vi "Close.vi"(0 "Data In":T2={"Console log"="", "GUI_Events"={"To_GUI-Producer"=refnum, "To_GUI-Error_message"=refnum, "To_GUI-msg_list"=refnum, "To_GUI-Session"=refnum, "To_GUI-Pre-Session"=refnum, "To_GUI-Consumer"=refnum}, "Function_Queue"={"Queue_MIDI_Handler"=refnum, "Queue_Session"=refnum, "Queue_Producer"=refnum, "Queue_Consumer"=refnum}, "Timout-Time[ms]"=0, "MIDI-Messages"=[], "Com Session State"=enum."Active Session", "Result Data"={"Diff"=[], "Tx Byte"=[], "Rx Byte"=[], "Send Log"=[], "Parsed Data"={"Tx MIDI Tag"=[], "Tx MIDI Parsed Data"=[], "Tx Error"=[], "Tx Running States"=[], "Rx MIDI Tag"=[], "Rx MIDI Parsed Data"=[], "Rx Error"=[], "Rx Running States"=[], "Diff"=[]}}, "Get #"=[], "CPU(ms)"=0}, 11 "Error In":errorcluster, 12 "MIDI Data":T19, 13 "Consumer Data":T15={"Queue_Consumer"=refnum, "Selected Consumer"=enum."Random", "Session Data"={"Tx-Data"=[], "Rx-Data"=[], "MIDI-Message log"=[{"Message Name"="", "Meta value"=0, "Datastring"="", "Datatype"=enum."No Data"}]}, "Timout-Time[ms]"=0, "To_GUI-Consumer"=refnum, "CPU(ms)"=0, "Console log"="", "MIDI Parse Data"={"MIDI-Bytes In"=[145, 60, 100], "MIDI Tag"=[], "MIDI Parsed Data"=[], "Iteration"=0, "Error?"=[], "Running States"=[], "Running Statusbyte"=0, "Running StatusString"="", "Third Byte Flag"=FALSE, "Current Byte"=0, "Sysex"="", "Expect Databyte"=FALSE}, "Session Inspection Data"={"Diff"=[], "Tx Byte"=[], "Rx Byte"=[], "Send Log"=[], "Parsed Data"={"Tx MIDI Tag"=[], "Tx MIDI Parsed Data"=[], "Tx Error"=[], "Tx Running States"=[], "Rx MIDI Tag"=[], "Rx MIDI Parsed Data"=[], "Rx Error"=[], "Rx Running States"=[], "Diff"=[]}}} {"MIDI Parse Data"."Current Byte" format="%.0x"; "MIDI Parse Data"."Running Statusbyte" format="%.0x"; "MIDI Parse Data"."MIDI-Bytes In" format="%.0x"}, 14 "Producer-Data":T11={"Queue_Producer"=refnum, "Queue_Consumer"=refnum, "To_GUI-Error_message"=refnum, "Rx-Data"=[], "Tx-Data"=[], "Console log"="", "Communication Settings"={"Tx Protocol"=enum."Not Active", "Rx Protocol"=enum."Serial", "Serial"={"Tx Port"="", "Rx Port"="", "Baud rate"=31250, "Parity"=enum."Space", "Data bits"=8, "Stop bits"=10, "Flow control"=enum."None", "Tx Resource"="", "Rx Resource"=""}, "MIDI Device"={"Input uDevice ID"=0, "Output uDevice ID"=0, "hmidiout Handle"=0, "hmidiin Handle"=0}, "Bluetooth"={"Dummy"=""}, "USB"={"Dummy"=""}}, "MIDI-Messages"=[], "Queue_Session"=refnum, "To_GUI-Pre-Session"=refnum, "To_GUI-Producer"=refnum, "Tx Info"={"Datatype"=[], "Bytesize"=[], "Strings"=[], "ByteSum"=0}, "Payload"=variant, "Timout-Time[ms]"=0, "To_GUI-Session"=refnum, "CPU(ms)"=0}) -> (15 "Error Out":errorcluster)   [LabVIEW 2019]
doc: "Closing of the software:\n- Storing console entries for debugging."
uses:
  Common/Controls/Application_Data.ctl
  Common/Controls/App_Events.ctl
  Common/Controls/App_Queues.ctl
  Common/Controls/Application_Message.ctl
  Common/Controls/Application_State.ctl
  MIDI/Controls/MIDI-Message_Array.ctl
  MIDI/Controls/MIDI-Message_Cluster.ctl
  MIDI/Controls/Meta_Commands.ctl
  Producer/Controls/Session_State.ctl
  Consumer/Controls/Consumer_Result.ctl
  Consumer/Controls/Parsed_Data.ctl
  Producer/Controls/Producer-Data.ctl
  Common/Controls/Communication_Settings.ctl
  Common/Controls/Communication_Protocols.ctl
  Producer/Controls/Prod - Tx_Info.ctl
  Consumer/Controls/Consumer_Data.ctl
  Consumer/Controls/Consumer_States.ctl
  Consumer/Controls/Transfer_Data.ctl
  Consumer/Controls/Parser-data.ctl
  MIDI/Controls/MIDI-Data.ctl
  <vilib>/Utility/error.llb/DialogType.ctl
  86581a33-42cb-4fee-adae-e4a703b4ff76.vi
  <vilib>/Array/Sort 2D Array - Pop Stack.vi
  <vilib>/Array/Sort 2D Array - Push Stack.vi
panel:
  in  "Tab Control":T1(tab)
  out "Final Console":string
  out "Error Message":string
  out "VI-filename":string
  out "VI Path":path
  in  "Tabs Visible?":bool
  in  "Tool Bar:Visible":bool
  out "Revision Number":u32
  out "VI-Name":string
  # "Settings"
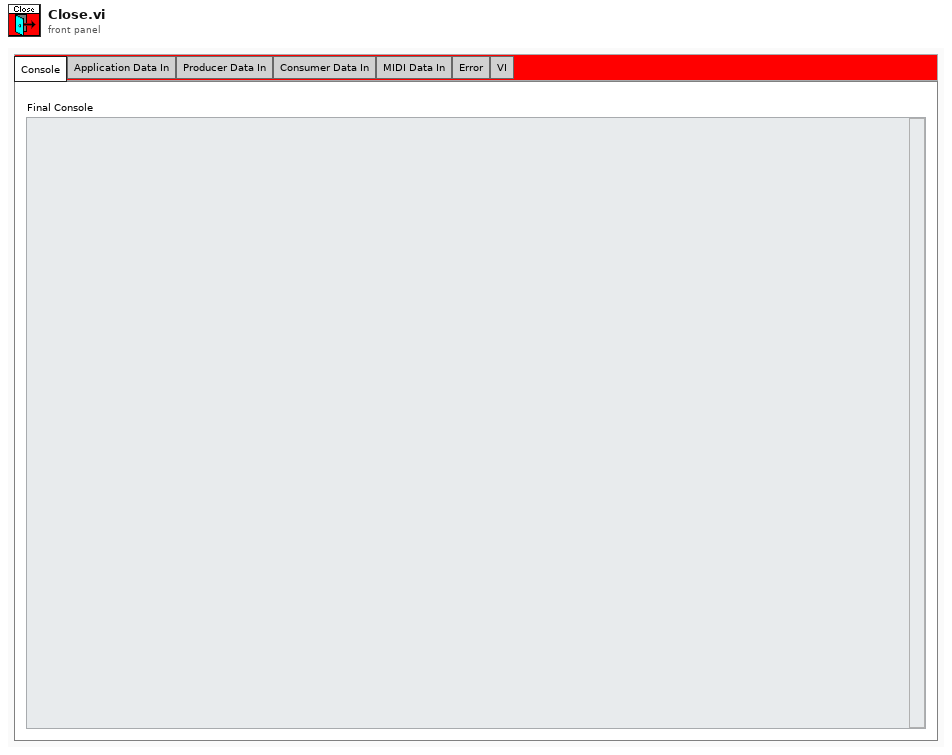
[diagram p1: front panel]
types:
  T1 = enum32{"Console", "Application Data In", "Producer Data In", "Consumer Data In", "MIDI Data In", "Error", "VI"}
  T2 = typedef "Application_Data.ctl" = cluster{"Console log":string, "GUI_Events":T3, "Function_Queue":T4, "Timout-Time[ms]":i32, "MIDI-Messages":T5, "Com Session State":T8, "Result Data":T9, "Get #":bool[], "CPU(ms)":u32}
  T3 = typedef "App_Events.ctl" = cluster{"To_GUI-Producer":refnum<user-event>, "To_GUI-Error_message":refnum<user-event>, "To_GUI-msg_list":refnum<user-event>, "To_GUI-Session":refnum<user-event>, "To_GUI-Pre-Session":refnum<user-event>, "To_GUI-Consumer":refnum<user-event>}
  T4 = typedef "App_Queues.ctl" = cluster{"Queue_MIDI_Handler":refnum<queue>, "Queue_Session":refnum<queue>, "Queue_Producer":refnum<queue>, "Queue_Consumer":refnum<queue>}
  T5 = typedef "MIDI-Message_Array.ctl" = T6[]
  T6 = typedef "MIDI-Message_Cluster.ctl" = cluster{"Message Name":string, "Meta value":i32, "Datastring":string, "Datatype":T7}
  T7 = typedef "Meta_Commands.ctl" = enum16{"No Data", "Pause", "Loop", "Wait for Rx", "Delay", "Break", "MIDI"}
  T8 = typedef "Session_State.ctl" = enum16{"Wait to begin", "Active Session", "Pause", "Wait for Response", "Stop", "Restart", "Inspect", "Exit"}
  T9 = typedef "Consumer_Result.ctl" = cluster{"Diff":bool[], "Tx Byte":string[], "Rx Byte":string[], "Send Log":string[], "Parsed Data":T10}
  T10 = typedef "Parsed_Data.ctl" = cluster{"Tx MIDI Tag":string[], "Tx MIDI Parsed Data":string[], "Tx Error":bool[], "Tx Running States":string[], "Rx MIDI Tag":string[], "Rx MIDI Parsed Data":string[], "Rx Error":bool[], "Rx Running States":string[], "Diff":bool[]}
  T11 = typedef "Producer-Data.ctl" = cluster{"Queue_Producer":refnum<queue>, "Queue_Consumer":refnum<queue>, "To_GUI-Error_message":refnum<user-event>, "Rx-Data":i8[], "Tx-Data":i8[], "Console log":string, "Communication Settings":T12, "MIDI-Messages":T5, "Queue_Session":refnum<queue>, "To_GUI-Pre-Session":refnum<user-event>, "To_GUI-Producer":refnum<user-event>, "Tx Info":T14, "Payload":variant, "Timout-Time[ms]":i32, "To_GUI-Session":refnum<user-event>, "CPU(ms)":u32}
  T12 = typedef "Communication_Settings.ctl" = cluster{"Tx Protocol":T13, "Rx Protocol":T13, "Serial":cluster{"Tx Port":refnum<visa-resource-name>, "Rx Port":refnum<visa-resource-name>, "Baud rate":i32, "Parity":enum16{"None", "Odd", "Even", "Mark", "Space"}, "Data bits":i32, "Stop bits":i32, "Flow control":enum16{"None", "XON/XOFF", "RTS/CTS", "XON/XOFF & RTS/CTS", "DTR/DSR", "XON/XOFF & DTR/DSR"}, "Tx Resource":refnum<visa-resource-name>, "Rx Resource":refnum<visa-resource-name>}, "MIDI Device":cluster{"Input uDevice ID":u32, "Output uDevice ID":u32, "hmidiout Handle":i32, "hmidiin Handle":i32}, "Bluetooth":cluster{"Dummy":string}, "USB":cluster{"Dummy":string}}
  T13 = typedef "Communication_Protocols.ctl" = enum16{"Serial", "Bluetooth", "USB-MIDI", "MIDI (Audio Device)", "Not Active"}
  T14 = typedef "Prod - Tx_Info.ctl" = cluster{"Datatype":T7[], "Bytesize":i32[], "Strings":string[], "ByteSum":i32}
  T15 = typedef "Consumer_Data.ctl" = cluster{"Queue_Consumer":refnum<queue>, "Selected Consumer":T16, "Session Data":T17, "Timout-Time[ms]":i32, "To_GUI-Consumer":refnum<user-event>, "CPU(ms)":u32, "Console log":string, "MIDI Parse Data":T18, "Session Inspection Data":T9}
  T16 = typedef "Consumer_States.ctl" = enum16{"Random", "ECG", "Strech-Patch"}
  T17 = typedef "Transfer_Data.ctl" = cluster{"Tx-Data":i8[], "Rx-Data":i8[], "MIDI-Message log":T5}
  T18 = typedef "Parser-data.ctl" = cluster{"MIDI-Bytes In":u8[], "MIDI Tag":string[], "MIDI Parsed Data":string[], "Iteration":i32, "Error?":bool[], "Running States":string[], "Running Statusbyte":u8, "Running StatusString":string, "Third Byte Flag":bool, "Current Byte":u8, "Sysex":string, "Expect Databyte":bool}
  T19 = typedef "MIDI-Data.ctl" = cluster{"Console log":string, "Payload":variant, "MIDI Message Array":T5, "Timout-Time[ms]":i32, "Queue_MIDI_Handler":refnum<queue>, "To_GUI-Error_message":refnum<user-event>, "To_GUI-msg_list":refnum<user-event>, "CPU(ms)":u32}
  T20 = enum16{"open", "replace", "create", "open or create", "replace or create", "replace or create with confirmation"}
  T21 = typedef "DialogType.ctl" = u16
  T22 = typedef "LVRectTypeDef.ctl" = cluster{"Left":i16, "Top":i16, "Right":i16, "Bottom":i16}
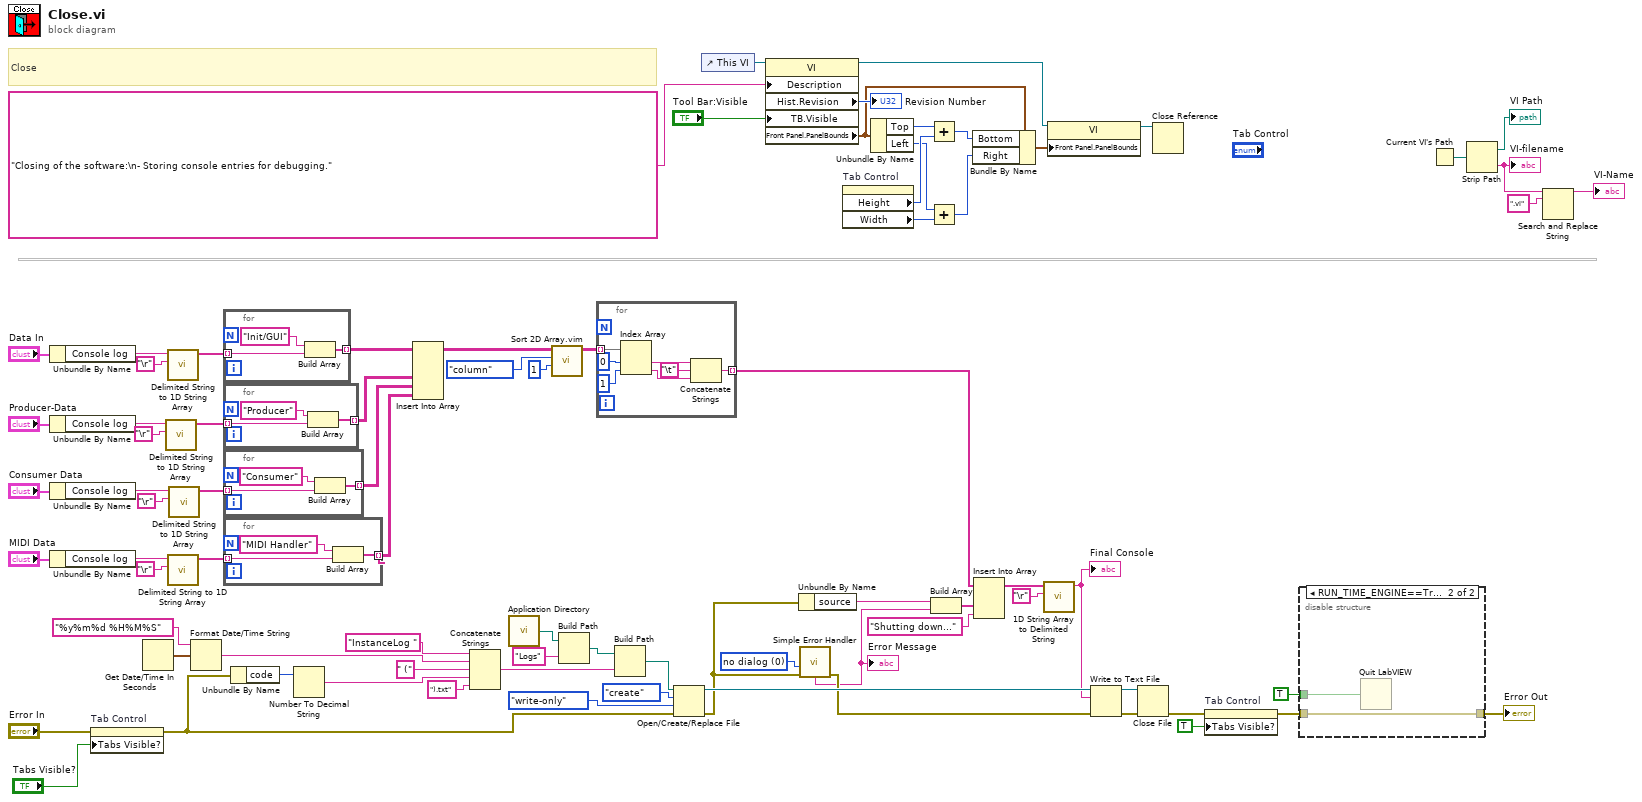
[diagram p0: block diagram]
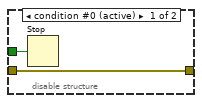
[diagram p2: hidden frame]
diagram:
  w46 = T21 0 items=["no dialog", "OK message", "continue or stop message", "OK message + warnings", "continue/stop + warnings"] ("type of dialog (OK msg:1)")
  # "Close"
  n1 = Unbundle By Name("Data In") -> ("Console log"=w62:string)
  n2 = Unbundle By Name("Producer-Data") -> ("Console log"=w61:string)
  n3 = Unbundle By Name("Consumer Data") -> ("Console log"=w60:string)
  n4 = Unbundle By Name("MIDI Data") -> ("Console log"=w67:string)
  n5 = property on="Tab Control" class="TabCtl (strict)"(error in="Error In", "Tabs Visible?"="Tabs Visible?") -> (error out=w15:errorcluster)  [unwired: 1 in, 1 out]
  n6 = Get Date/Time In Seconds() -> (seconds since 1Jan1904=w55:timestamp)
  n7 = call <vilib>:"Delimited String to 1D String Array.vi"("delimiter"="\r", "delimited string"=w61) -> ("string array"=w42:string[])  [unwired: 9 in]
  n8 = call <vilib>:"Delimited String to 1D String Array.vi"("delimiter"="\r", "delimited string"=w62) -> ("string array"=w43:string[])  [unwired: 9 in]
  n9 = call <vilib>:"Delimited String to 1D String Array.vi"("delimiter"="\r", "delimited string"=w67) -> ("string array"=w40:string[])  [unwired: 9 in]
  n10 = call <vilib>:"Delimited String to 1D String Array.vi"("delimiter"="\r", "delimited string"=w60) -> ("string array"=w41:string[])  [unwired: 9 in]
  n11 = Format Date/Time String(time format string (%c)="%y%m%d %H%M%S", seconds (now)=w55) -> (date/time string=w53:string)  [unwired: 1 in]
  n12 = for {
    tunnel: w43 -> [w83] mode=indexing
    tunnel: [w82] -> w39 mode=indexing
    n13 = Build Array("Init/GUI" ("element"), w83) -> (w82:string[])
  }
  n14 = for {
    tunnel: w42 -> [w86] mode=indexing
    tunnel: [w85] -> w38 mode=indexing
    n15 = Build Array("Producer" ("element"), w86) -> (w85:string[])
  }
  n16 = for {
    tunnel: w41 -> [w89] mode=indexing
    tunnel: [w88] -> w37 mode=indexing
    n17 = Build Array("Consumer" ("element"), w89) -> (w88:string[])
  }
  n18 = for {
    tunnel: w40 -> [w92] mode=indexing
    tunnel: [w91] -> w36 mode=indexing
    n19 = Build Array("MIDI Handler" ("element"), w92) -> (w91:string[])
  }
  n20 = Unbundle By Name(w15) -> ("code"=w52:i32)
  n21 = Number To Decimal String(number=w52) -> (decimal integer string=w50:string)  [unwired: 1 in]
  n22 = Insert Into Array(array=w39, new element #1=w38, new element #2=w37, new element #3=w36) -> (w35:string[][])  [unwired: 2 in]
  n23 = Concatenate Strings("InstanceLog ", w53, " (" ("string"), w50, ").txt" ("string")) -> (w48:string)
  n24 = call <vilib>:"Application Directory.vi"() -> ("Application Directory"=w59:path)
  n25 = call "Sort 2D Array.vim"("index"=1, "dimension to index (column)"=enum16{"column", "row"}."column", "2D array"=w35) -> ("sorted 2D array"=w32:string[][])  [unwired: 7 in, 1 out]
  n26 = Build Path(base path=w59, name or relative path="Logs") -> (appended path=w57:path)
  n27 = for {
    tunnel: w32 -> [w99] mode=indexing
    tunnel: [w95] -> w24 mode=indexing
    n28 = Index Array(array=w99, index #1=0 ("index"), index #2=1 ("index")) -> (element #1=w98:string, element #2=w94:string)
    n29 = Concatenate Strings(w98, "\t", w94) -> (w95:string)
  }
  n30 = Build Path(base path=w57, name or relative path=w48) -> (appended path=w30:path)
  n31 = Open/Create/Replace File(file path (use dialog)=w30, error in=w15, operation (0:open)=T20."create", access (0:read/write)=enum16{"read/write", "read-only", "write-only"}."write-only") -> (refnum out=w27:refnum<file>, error out=w14:errorcluster)  [unwired: 2 in, 1 out]
  n32 = control-ref of="This VI"() -> (w11:refnum<vi>)
  n33 = property class="VI"(reference=w11, "Description"="Closing of the software:\n- Storing console entries for debugging.", "TB.Visible"="Tool Bar:Visible") -> (reference out=w8:refnum<vi>, "Hist.Revision"=→"Revision Number":u32, "Front Panel.PanelBounds"=w7:T22)  [unwired: 1 in, 1 out]
  n34 = Unbundle By Name(w14) -> ("source"=w21:string)
  n35 = call <vilib>:"Simple Error Handler.vi"("type of dialog (OK msg:1)"=w46, "error in (no error)"=w14) -> ("error out"=w22:errorcluster, "message"=w20:string)  [unwired: 3 in, 3 out]
  "Error Message" <- w20
  n36 = property on="Tab Control" class="TabCtl (strict)"() -> ("Height"=w9:u32, "Width"=w2:u32)  [unwired: 2 in, 2 out]
  n37 = Unbundle By Name(w7) -> ("Top"=w10:i16, "Left"=w3:i16)
  n38 = Add(x=w10, y=w9) -> (x+y=w6:u32)
  n39 = Add(x=w3, y=w2) -> (x+y=w4:u32)
  n40 = Build Array(w21, w20) -> (w19:string[])
  n41 = Bundle By Name(cluster=w7, "Bottom"=w6, "Right"=w4) -> (w5:T22)
  n42 = Insert Into Array(array=w24, new element #1=w19, new element #2="Shutting down..." ("new element/subarray")) -> (w23:string[])  [unwired: 1 in]
  n43 = call <vilib>:"1D String Array to Delimited String.vi"("delimiter"="\r", "string array"=w23) -> ("delimited string"=w17:string)  [unwired: 9 in]
  "Final Console" <- w17
  n44 = property class="VI"(reference=w8, "Front Panel.PanelBounds"=w5) -> (reference out=w1:refnum<vi>)  [unwired: 1 in, 1 out]
  n45 = Write to Text File(file (use dialog)=w27, text=w17, error in=w22) -> (refnum out=w25:refnum<file>, error out=w26:errorcluster)  [unwired: 1 in, 1 out]
  n46 = Close File(refnum=w25, error in=w26) -> (error out=w13:errorcluster)  [unwired: 1 out]
  n47 = Close Reference(reference=w1) -> ()  [unwired: 1 in, 1 out]
  n48 = property on="Tab Control" class="TabCtl (strict)"(error in=w13, "Tabs Visible?"=TRUE) -> (error out=w12:errorcluster)  [unwired: 1 in, 1 out]
  n49 = disable-structure "Conditional Disable Structure" shown="RUN_TIME_ENGINE==True" {
    disable-tunnel: TRUE ("stop? (T)") -> [w101 w103]
    disable-tunnel: w12 -> [w100 w102]
    disable-tunnel: [w100 w102] -> w44
    frame condition #0 (active) {
      n50 = Stop(stop? (T)=w101) -> ()
    }
    frame condition #1 {
      n51 = Quit LabVIEW(quit? (T)=w103) -> ()
    }
  }
  "Error Out" <- w44
  n52 = Current VI's Path() -> (path=w80:path)
  n53 = Strip Path(path=w80) -> (stripped path=→"VI Path":path, name=w75:string)
  "VI-filename" <- w75
  n54 = Search and Replace String(input string=w75, search string=".vi") -> (result string=→"VI-Name":string)  [unwired: 6 in, 3 out]
